vi "Configure Branch Limit Constant.vi"(0 "VISA resource name":refnum<visa-resource-name>, 1 "Limit B (0)":dbl, 2 "Measure Block (0)":u32, 5 "Block Number (1)":u32=1, 7 "Limit Type (0)":i32(ring) items=["Above", "Below", "Inside", "Outside"], 9 "Limit A (0)":dbl, 11 "error in (no error)":errorcluster, 12 "Branch To Block (0)":u32) -> (4 "VISA resource name out":refnum<visa-resource-name>, 15 "error out":errorcluster)   [LabVIEW 2015, in "Keithley DMM6500 DAQ6500 Series.lvlib"]
doc: "Defines a trigger model block that goes to a specified block if a measurement meets preset criteria."
uses:
  <instrlib>/Keithley DMM6500 DAQ6500 Series/Keithley DMM6500 DAQ6500 Series.lvlib
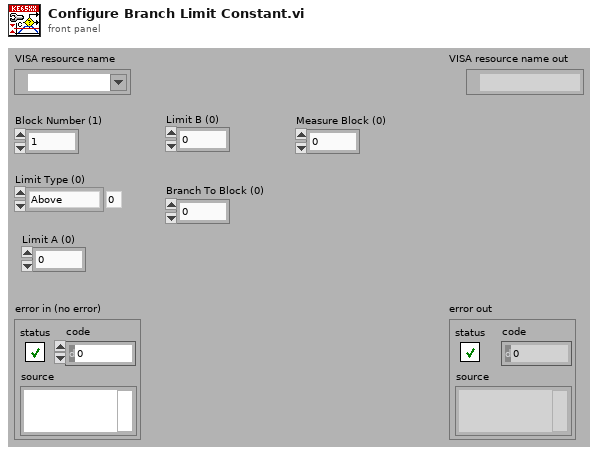
[diagram p1: front panel]
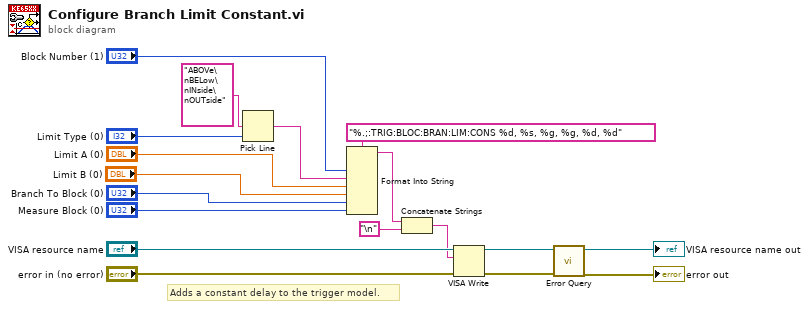
[diagram p0: block diagram]
diagram:
  # "Adds a constant delay to the trigger model."
  n1 = Pick Line(multi-line string="ABOVe\nBELow\nINside\nOUTside", line index="Limit Type (0)") -> (output string=w9:string)  [unwired: 1 in]
  n2 = Format Into String(format string="%.;:TRIG:BLOC:BRAN:LIM:CONS %d, %s, %g, %g, %d, %d", "Block Number (1)", w9, "Limit A (0)", "Limit B (0)", "Branch To Block (0)", "Measure Block (0)") -> (resulting string=w2:string)  [unwired: 2 in, 1 out]
  n3 = Concatenate Strings(w2, "\n") -> (w3:string)
  n4 = VISA Write(VISA resource name="VISA resource name", write buffer=w3, error in (no error)="error in (no error)") -> (VISA resource name out=w15:refnum<visa-resource-name>, error out=w14:errorcluster)  [unwired: 1 out]
  n5 = call <instrlib>:"Error Query.vi"("error in (no error)"=w14, "VISA resource name"=w15) -> ("error out"=→"error out":errorcluster, "VISA resource name out"=→"VISA resource name out":refnum<visa-resource-name>)  [unwired: 6 in, 2 out]
